vi "TPI set freq.vi"(8 "Error in (no error)":errorcluster, 9 "set freq (kHz)":u32=350000, 11 "VISA resource name":refnum<visa-resource-name>) -> (0 "Error out":errorcluster, 3 "VISA resource name out":refnum<visa-resource-name>)   [LabVIEW 2020]
panel:
  # "freq must be between 35000 kHz and 4400000 kHz inclusive\nVI coerces freq to be in this range"
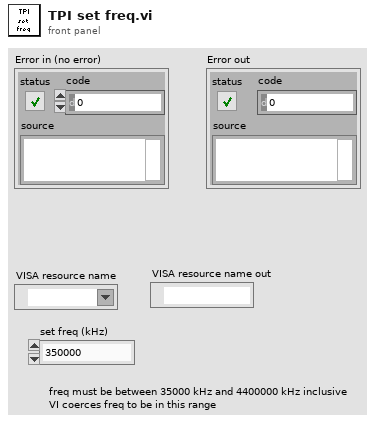
[diagram p1: front panel]
types:
  T1 = enum16{"big-endian, network order", "native, host order", "little-endian"}
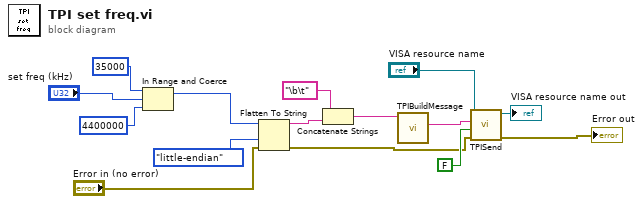
[diagram p0: block diagram]
diagram:
  n1 = In Range and Coerce(upper limit=u32 35000, x="set freq (kHz)", lower limit=u32 4400000 ("upper limit")) -> (coerced(x)=w7:u32)  [unwired: 1 out]
  n2 = Flatten To String(anything=w7, byte order (0:big-endian, network order)=T1."little-endian", error in (no error)="Error in (no error)") -> (data string=w14:string, error out=w2:errorcluster)  [unwired: 1 in, 1 out]
  n3 = Concatenate Strings("\b\t" ("Command"), w14) -> (w10:string)
  n4 = call "TPIBuildMessage.vi"("Command"=w10) -> ("Message"=w11:string)  [unwired: 10 in]
  n5 = call "TPISend.vi"("error in (no error)"=w2, "Read Responce"=FALSE, "write buffer"=w11, "VISA resource name"="VISA resource name") -> ("error out"=→"Error out":errorcluster, "VISA resource name out"=→"VISA resource name out":refnum<visa-resource-name>)  [unwired: 5 in, 1 out]
